vi "Nfocus driver V0.1.vi"(8 "Refs In":T1) -> (0 "error out":errorcluster)   [LabVIEW 2016]
panel:
  in  "error in":errorcluster
  out "Running":bool
  out "RelativeMove":dbl
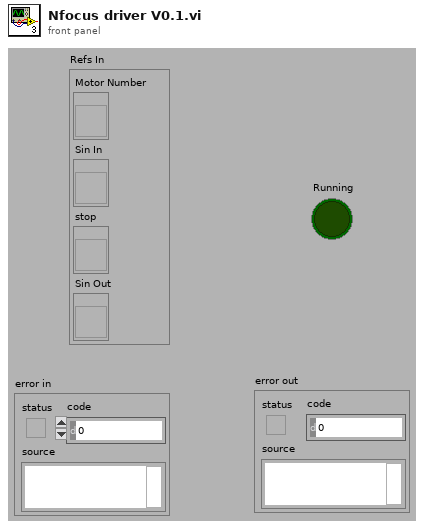
[diagram p1: front panel]
types:
  T1 = cluster{"Motor Number":refnum<vi>, "Sin In":refnum<vi>, "stop":refnum<vi>, "Sin Out":refnum<vi>}
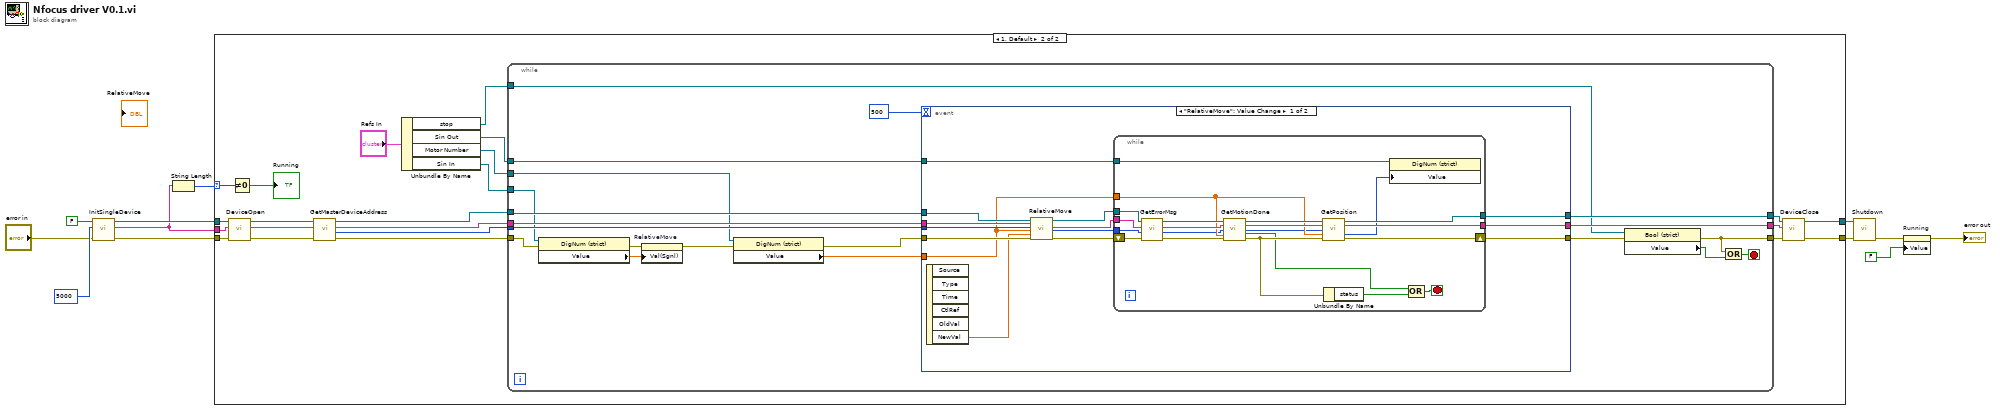
[diagram p0: block diagram]
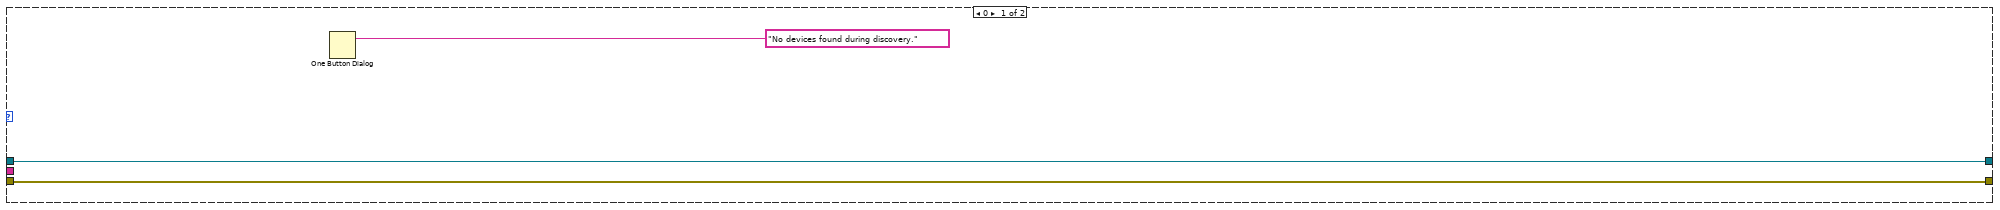
[diagram p2: hidden frame]
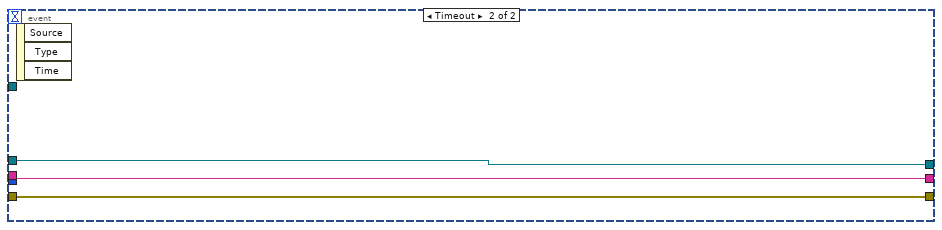
[diagram p3: hidden frame]
diagram:
  n1 = call "InitSingleDevice.vi"("error in (no error)"="error in", "msecDelayForDiscovery"=5000, "logging"=FALSE) -> ("error out"=w5:errorcluster, "DeviceKey Out"=w6:string, "CmdLib Out"=w8:refnum<k24>)  [unwired: 2 in]
  n2 = String Length(string=w6) -> (length=w7:i32)
  n3 = case shown="1, Default" w7 {
    selector: w7 -> [_ w22]
    tunnel: [w14 w24] -> w10
    tunnel: [w13 w26] -> w9
    tunnel: w8 -> [w14 w30]
    tunnel: w6 -> [_ w32]
    tunnel: w5 -> [w13 w34]
    frame 0 {
      n4 = One Button Dialog(message="No devices found during discovery.") -> ()  [unwired: 1 in, 1 out]
    }
    frame 1, Default {
      n5 = call "DeviceOpen.vi"("error in (no error)"=w34, "DeviceKey In"=w32, "CmdLib In"=w30) -> ("error out"=w33:errorcluster, "DeviceKey Out"=w31:string, "CmdLib Out"=w29:refnum<k24>)  [unwired: 2 in]
      n6 = Not Equal To 0?(x=w22) -> (x != 0?=→"Running":bool)
      n7 = call "GetMasterDeviceAddress.vi"("error in (no error)"=w33, "DeviceKey In"=w31, "CmdLib In"=w29) -> ("error out"=w23:errorcluster, "Device Address"=w37:i32, "DeviceKey Out"=w35:string, "CmdLib Out"=w36:refnum<k24>)  [unwired: 1 in]
      n8 = Unbundle By Name("Refs In") -> ("stop"=w16:refnum<vi>, "Sin Out"=w17:refnum<vi>, "Motor Number"=w19:refnum<vi>, "Sin In"=w18:refnum<vi>)
      n9 = while {
        tunnel: w37 -> [w57]
        tunnel: w36 -> [w56]
        tunnel: [w53] -> w25
        tunnel: w23 -> [w52]
        tunnel: [w45] -> w27
        tunnel: w35 -> [w55]
        tunnel: [w54] -> w28
        tunnel: w18 -> [w40]
        tunnel: w19 -> [w38]
        tunnel: w17 -> [w42]
        tunnel: w16 -> [w41]
        stop <- w47 stop-if-true
        n10 = property on="Property Node" class="DigNum (strict)"(reference=w40, error in=w52) -> (error out=w48:errorcluster, "Value"=w49:sgl)  [unwired: 1 out]
        n11 = property on="RelativeMove" class="DigNum (strict)"(error in=w48, "Val(Sgnl)"=w49) -> (error out=w39:errorcluster)  [unwired: 1 in, 1 out]
        n12 = property on="Property Node" class="DigNum (strict)"(reference=w38, error in=w39) -> (error out=w51:errorcluster, "Value"=w50:dbl)  [unwired: 1 out]
        n13 = event shown="[0] \"RelativeMove\": Value Change" {
          selector: _ -> [_ _]
          dyn-events: _ -> [_ _]
          timeout: 500 -> [_ _]
          tunnel: w57 -> [w71 _]
          tunnel: w51 -> [w70 w93]
          tunnel: w56 -> [w69 w95]
          tunnel: w55 -> [w68 w94]
          tunnel: [w67 w94] -> w54
          tunnel: [w66 w93] -> w46
          tunnel: [w65 w95] -> w53
          tunnel: w50 -> [w59 _]
          tunnel: w42 -> [w58 _]
          event "RelativeMove": Value Change {
            n14 = event-data() -> ("NewVal"=w60:dbl)  [unwired: 1 in, 5 out]
            n15 = call "RelativeMove.vi"("CmdLib In"=w69, "DeviceKey In"=w68, "Device Address In"=w71, "Motor"=w59, "Relative Steps"=w60, "error in (no error)"=w70) -> ("CmdLib Out"=w64:refnum<k24>, "DeviceKey Out"=w63:string, "Device Address Out"=w61:i32, "error out"=w62:errorcluster)  [unwired: 10 in]
            n16 = while {
              tunnel: w59 -> [w88]
              tunnel: w64 -> [w87]
              tunnel: w63 -> [w86]
              tunnel: [w81] -> w65
              tunnel: w61 -> [w80]
              shift-right: [w82] -> w66
              shift-left: w62 -> [w85]
              tunnel: [w77] -> w67
              tunnel: w58 -> [w72]
              stop <- w76 stop-if-true
              n17 = call "GetErrorMsg.vi"("error in (no error)"=w85, "Device Address In"=w80, "DeviceKey In"=w86, "CmdLib In"=w87) -> ("error out"=w84:errorcluster, "Device Address Out"=w79:i32, "DeviceKey Out"=w90:string, "CmdLib Out"=w89:refnum<k24>)
              n18 = call "GetMotionDone.vi"("CmdLib In"=w89, "DeviceKey In"=w90, "Device Address In"=w79, "Motor"=w88, "error in (no error)"=w84) -> ("CmdLib Out"=w91:refnum<k24>, "DeviceKey Out"=w92:string, "Device Address Out"=w78:i32, "Is Motion Done"=w75:bool, "error out"=w83:errorcluster)  [unwired: 6 in]
              n19 = call "GetPosition.vi"("CmdLib In"=w91, "DeviceKey In"=w92, "Device Address In"=w78, "Motor"=w88, "error in (no error)"=w83) -> ("CmdLib Out"=w81:refnum<k24>, "DeviceKey Out"=w77:string, "Position"=w73:i32, "error out"=w82:errorcluster)  [unwired: 6 in, 1 out]
              n20 = Unbundle By Name(w83) -> ("status"=w74:bool)
              n21 = property on="Property Node" class="DigNum (strict)"(reference=w72, "Value"=w73) -> ()  [unwired: 1 in, 2 out]
              n22 = Compound Arithmetic op=OR(w75, w74) -> (w76:bool)
            }
          }
          event Timeout {
            n23 = event-data() -> ()  [unwired: 1 in, 3 out]
          }
        }
        n24 = property on="Property Node" class="Bool (strict)"(reference=w41, error in=w46) -> (error out=w45:errorcluster, "Value"=w44:bool)  [unwired: 1 out]
        n25 = Compound Arithmetic op=OR(w45, w44) -> (w47:bool)
      }
      n26 = call "DeviceClose.vi"("error in (no error)"=w27, "DeviceKey In"=w28, "CmdLib In"=w25) -> ("error out"=w26:errorcluster, "CmdLib Out"=w24:refnum<k24>)  [unwired: 2 in, 1 out]
    }
  }
  n27 = call "Shutdown.vi"("error in (no error)"=w9, "CmdLib In"=w10) -> ("error out"=w3:errorcluster)  [unwired: 4 in, 1 out]
  n28 = property on="Running" class="Bool (strict)"(error in=w3, "Value"=FALSE ("Boolean")) -> (error out=→"error out":errorcluster)  [unwired: 1 in, 1 out]
